vi "VCS Get Driver Info.vi"(11 "error in (no error)":errorcluster) -> (4 "libraryName":string, 6 "libraryVersion":string, 15 "error out":errorcluster)   [LabVIEW 2017, in "maxonEPOS.lvlib"]
doc: "<B>VCS Get Driver Info</B> returns the name and version from the Windows DLL."
uses:
  Examples/maxonEPOS.lvlib
  Resources/EposCmd.dll
  SSI_Tool/InstrumentsInterfaces/Motordriver/maxon EPOS/Resources/EposCmd64.dll
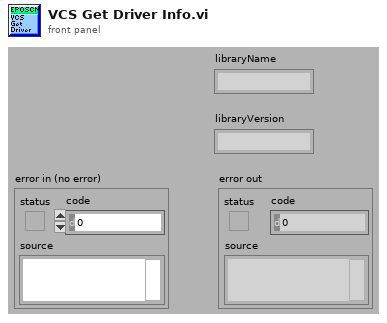
[diagram p1: front panel]
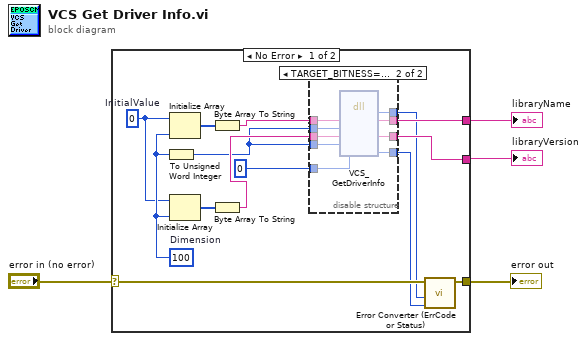
[diagram p0: block diagram]
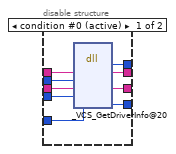
[diagram p2: hidden frame]
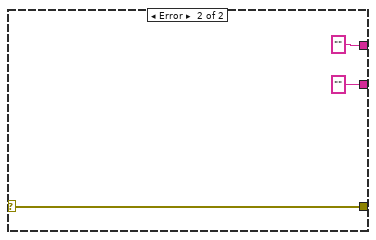
[diagram p3: hidden frame]
diagram:
  n1 = case shown="No Error" "error in (no error)" {
    selector: "error in (no error)" -> [w16 w39]
    tunnel: [w15 w39] -> w3
    tunnel: [w18 "" ("pLibraryName")] -> w2
    tunnel: [w17 "" ("pLibraryVersion")] -> w1
    frame No Error {
      w5 = u8 0  # InitialValue
      w6 = 100  # Dimension
      n2 = To Unsigned Word Integer(number=w6) -> (unsigned 16bit integer=w7:u16)
      n3 = Initialize Array(w5, w6) -> (w12:u8[])
      n4 = Initialize Array(w5, w6) -> (w13:u8[])
      n5 = Byte Array To String(unsigned byte array=w12) -> (string=w11:string)
      n6 = Byte Array To String(unsigned byte array=w13) -> (string=w10:string)
      n7 = disable-structure shown="TARGET_BITNESS==64" {
        disable-tunnel: [w27 w36] -> w18
        disable-tunnel: [w26 w35] -> w17
        disable-tunnel: [w25 w34] -> w14
        disable-tunnel: w11 -> [w24 w33]
        disable-tunnel: w7 -> [w23 w32]
        disable-tunnel: w10 -> [w22 w31]
        disable-tunnel: w7 -> [w21 w30]
        disable-tunnel: u32 0 ("pErrorCode") -> [w20 w29]
        disable-tunnel: [w19 w28] -> w8
        frame condition #0 (active) {
          n8 = dll-call lib="C:/workspace/project/scancon/sw/SSI_Tool/InstrumentsInterfaces/Motordriver/maxon EPOS/Resources/EposCmd.*" fn="_VCS_GetDriverInfo@20"("pLibraryName"=w24, "MaxStrNameSize"=w23, "pLibraryVersion"=w22, "MaxStrVersionSize"=w21, "pErrorCode"=w20) -> (w19:i32, "pLibraryName"=w27:string, "pLibraryVersion"=w26:string, "pErrorCode"=w25:u32)  [unwired: 5 in, 2 out]
        }
        frame condition #1 {
          n9 = dll-call lib="C:/Sources/LabView/maxon EPOS/Resources/EposCmd64.*" fn="VCS_GetDriverInfo" ("EposCmd.dll:_VCS_GetDriverInfo@20")("pLibraryName"=w33, "MaxStrNameSize"=w32, "pLibraryVersion"=w31, "MaxStrVersionSize"=w30, "pErrorCode"=w29) -> ("Rückgabetyp"=w28:i32, "pLibraryName"=w36:string, "pLibraryVersion"=w35:string, "pErrorCode"=w34:u32)  [unwired: 5 in, 2 out]
        }
      }
      n10 = call "Error Converter (ErrCode or Status).vi"("error code"=w14, "return type"=w8, "error in (no error)"=w16) -> ("error out"=w15:errorcluster)  [unwired: 7 in]
    }
    frame Error {
    }
  }
  "libraryName" <- w2
  "libraryVersion" <- w1
  "error out" <- w3
